vi "Counter Launcher.vi"(9 "Sub Panel":refnum<vi>, 10 "Counter ID":string="Secondary", 11 "Feeder Actor In":refnum<class "Feeder.lvclass">) -> (2 "Nested Actor's Enqueuer":refnum<class "Message Enqueuer.lvclass">, 3 "Feeder Actor Out":refnum<class "Feeder.lvclass">)   [LabVIEW 2018, in "Feeder Actor.lvlib" / "Counter.lvclass"]
uses:
  Counter.lvclass
  Feeder/Feeder.lvclass
  C:/Program Files/National Instruments/LabVIEW 2018/vi.lib/MGI/Panel Manager/Panel Actor/Panel Actor/Panel Actor.lvclass
  <vilib>/ActorFramework/Message Enqueuer/Message Enqueuer.lvclass
  Counter.lvclass/Counter.ctl
  <vilib>/MGI/Panel Manager/Panel/Panel/Subpanel/Subpanel.lvclass
  C:/Program Files/National Instruments/LabVIEW 2018/vi.lib/MGI/Panel Manager/Panel/Panel/Panel.lvclass
  <vilib>/DAQmx/create/channels.llb/DAQmx Create Channel (CO-Pulse Generation-Frequency).vi
  <vilib>/MGI/Panel Manager/Panel/Panel/Subpanel/Subpanel.vi
  <vilib>/DAQmx/configure/timing.llb/DAQmx Timing (Implicit).vi
  <vilib>/MGI/Panel Manager/Panel/Panel.lvlib
  <vilib>/MGI/Panel Manager/Panel Actor/Panel Actor/Panel Actor.lvclass
  ADM/Main.lvlib
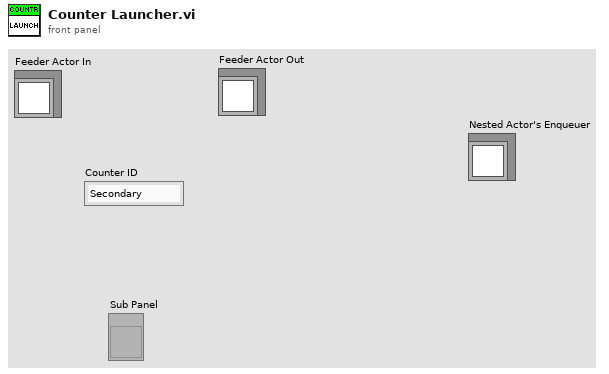
[diagram p1: front panel]
types:
  T1 = cluster{"Task Name":string, "Task Type":enum16{"VISA", "DAQmx"}, "VISA Resource Name":refnum<visa-resource-name>, "DAQmx Channel Name":tag}
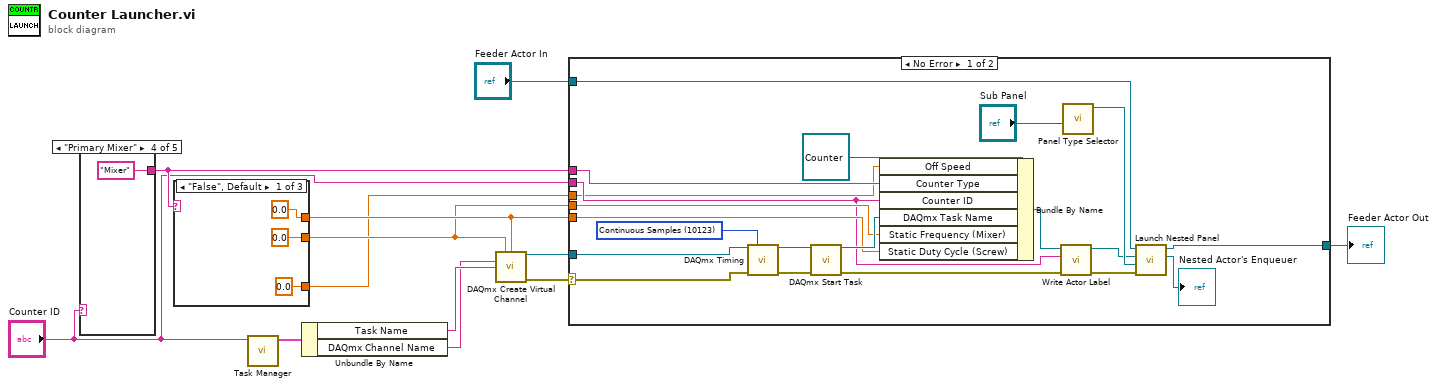
[diagram p0: block diagram]
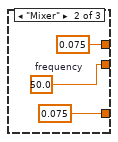
[diagram p2: hidden frame]
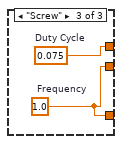
[diagram p3: hidden frame]
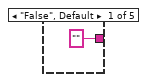
[diagram p4: hidden frame]
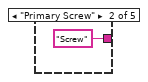
[diagram p5: hidden frame]
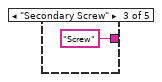
[diagram p6: hidden frame]
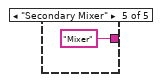
[diagram p7: hidden frame]
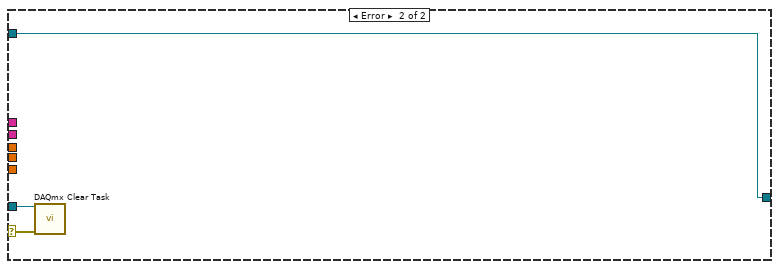
[diagram p8: hidden frame]
diagram:
  n1 = case shown="\"Primary Mixer\"" "Counter ID" {
    tunnel: ["" "Screw" "Screw" "Mixer" "Mixer"] -> w6
    frame "False", Default {
    }
    frame "Primary Screw" {
    }
    frame "Secondary Screw" {
    }
    frame "Primary Mixer" {
    }
    frame "Secondary Mixer" {
    }
  }
  n2 = case shown="\"False\", Default" w6 {
    tunnel: [0.0 ("Duty Cycle") 0.075 ("duty cycle") w25] -> w8
    tunnel: [0.0 ("Frequency") w22 w24] -> w7
    tunnel: [0.0 ("Frequency") 0.075 w24] -> w1
    frame "False", Default {
    }
    frame "Mixer" {
      w22 = 50.0  # frequency
    }
    frame "Screw" {
      w24 = 1.0  # Frequency
      w25 = 0.075  # Duty Cycle
    }
  }
  n3 = call "Task Manager.vi"("Task"="Counter ID") -> ("Task Properties"=w4:T1)  [unwired: 9 in, 1 out]
  n4 = Unbundle By Name(w4) -> ("Task Name"=w3:string, "DAQmx Channel Name"=w2:tag)
  n5 = call-poly <vilib>:"DAQmx Create Virtual Channel.vi"("frequency"=w7, "duty cycle"=w8, "counter"=w2, "name to assign"=w3) -> ("task out"=w9:refnum<k21>, "error out"=w10:errorcluster)  [unwired: 10 in]
  n6 = case shown="No Error" w10 {
    selector: w10 -> [w40 w47]
    tunnel: "Feeder Actor In" -> [w32 w49]
    tunnel: [w43 w49] -> w11
    tunnel: w9 -> [w39 w48]
    tunnel: w7 -> [w37 _]
    tunnel: w8 -> [w36 _]
    tunnel: "Counter ID" -> [w29 _]
    tunnel: w6 -> [w33 _]
    tunnel: w1 -> [w26 _]
    frame No Error {
      w35 = 10123 items=["Finite Samples"=10178, "Continuous Samples"=10123, "Hardware Timed Single Point"=12522] ("sample mode")
      n7 = call-poly <vilib>:"DAQmx Timing.vi"("task/channels in"=w39, "sample mode"=w35, "error in"=w40) -> ("task out"=w42:refnum<k21>, "error out"=w41:errorcluster)  [unwired: 11 in]
      n8 = call <vilib>:"DAQmx Start Task.vi"("task/channels in"=w42, "error in"=w41) -> ("task out"=w38:refnum<k21>, "error out"=w28:errorcluster)  [unwired: 12 in]
      n9 = Bundle By Name(cluster=refnum<class "Counter.lvclass"> refnum ("Feeder Actor.lvlib:Counter.lvclass"), "Off Speed"=w26, "Counter Type"=w33, "Counter ID"=w29, "DAQmx Task Name"=w38, "Static Frequency (Mixer)"=w37, "Static Duty Cycle (Screw)"=w36) -> (w31:refnum<class "Counter.lvclass">)
      n10 = call-dynamic "Write Actor Label.vi"("error in (no error)"=w28, "Actor Label"=w29, "Monitored Actor in"=w31) -> ("error out"=w27:errorcluster, "Monitored Actor out"=w30:refnum<class "Counter.lvclass">)  [unwired: 7 in]
      n11 = call-poly <vilib>:"Panel Type Selector.vi"("Sub Panel"="Sub Panel") -> ("Subpanel Out"=w44:refnum<class "Subpanel.lvclass">)  [unwired: 9 in, 1 out]
      n12 = call <vilib>:"Launch Nested Panel.vi"("error in (no error)"=w27, "Panel"=w44, "Nested Panel Actor"=w30, "Panel Actor in"=w32) -> ("Nested Actor's Enqueuer"=→"Nested Actor's Enqueuer":refnum<class "Message Enqueuer.lvclass">, "Panel Actor out"=w43:refnum<class "Feeder.lvclass">)  [unwired: 4 in, 2 out]
    }
    frame Error {
      n13 = call <vilib>:"DAQmx Clear Task.vi"("task in"=w48, "error in"=w47) -> ()  [unwired: 13 in, 1 out]
    }
  }
  "Feeder Actor Out" <- w11
